vi "Stitch DAQ-scope data.vi"(0 "DAQ time array (decimated)":dbl[](array[numeric]), 5 "DAQ DOD (final)":dbl[](array[numeric]), 7 "Scope Time arrays.Time axis":dbl[](array[numeric]), 9 "Scope Data arrays.CH1 (final A-B)":dbl[](array[numeric]), 11 "error in":errorcluster) -> (4 ">> max scope time":dbl, 6 "Stitched data array":dbl[](array[numeric]), 15 "error out":errorcluster)   [LabVIEW 2017, in "Processing.lvlib"]
uses:
  Processing.lvlib
  <vilib>/Analysis/baseanly.llb/Mean (DBL).vi
  <vilib>/Analysis/NI_AALBase.lvlib
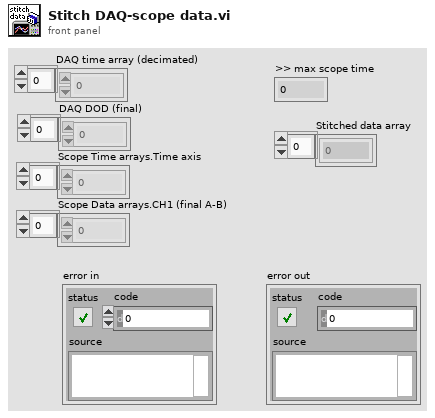
[diagram p1: front panel]
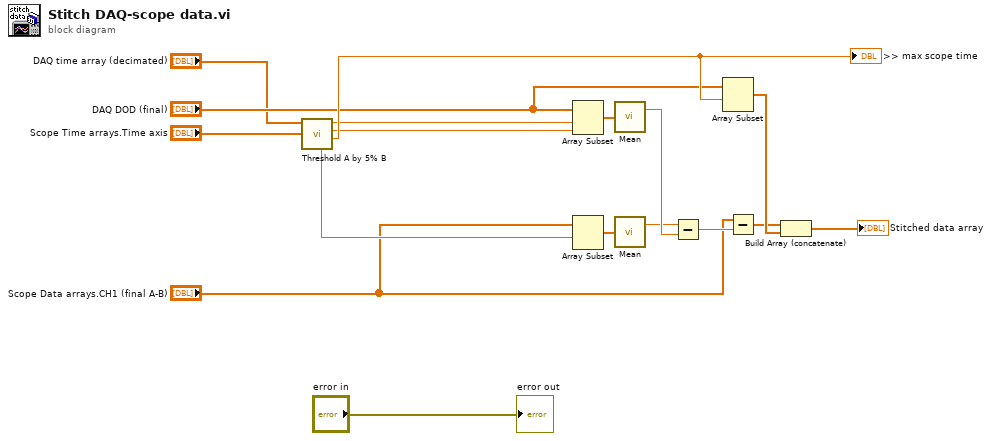
[diagram p0: block diagram]
diagram:
  n1 = call "Threshold A by 5% B.vi"("array B"="Scope Time arrays.Time axis", "array A"="DAQ time array (decimated)") -> ("Where array B = 100% of array A"=w17:dbl, "threshold difference"=w14:dbl, "Where array B = 95% of array A"=w15:dbl, "index of 95% of array A"=w16:dbl)  [unwired: 6 in]
  ">> max scope time" <- w17
  n2 = Array Subset(array="DAQ DOD (final)", index=w15, length=w14) -> (w7:dbl[])
  n3 = Array Subset(array="Scope Data arrays.CH1 (final A-B)", index=w16) -> (w6:dbl[])  [unwired: 1 in]
  n4 = call-poly <vilib>:"Mean.vi"("X"=w7) -> ("mean"=w10:dbl)  [unwired: 1 out]
  n5 = call-poly <vilib>:"Mean.vi"("X"=w6) -> ("mean"=w9:dbl)  [unwired: 1 out]
  n6 = Subtract(x=w9, y=w10) -> (x-y=w8:dbl)
  n7 = Array Subset(array="DAQ DOD (final)", index=w17) -> (w12:dbl[])  [unwired: 1 in]
  n8 = Subtract(x="Scope Data arrays.CH1 (final A-B)", y=w8) -> (x-y=w11:dbl[])
  n9 = Build Array (concatenate)(w11, w12) -> (→"Stitched data array":dbl[])
  "error out" <- "error in"
